vi "ConfigureSsiAbsEncoderSensorType.vi"(4 "error in (no error)":errorcluster, 5 "SSI sensor type":u16(ring)=4 items=["SSI encoder binary coded"=4, "SSI encoder grey coded"=5], 6 "SSI encoder configuration":T1, 7 "axis in":cluster{"keyHandle":u32, "nodeId":u16}={"keyHandle"=0, "nodeId"=1}) -> (0 "error out":errorcluster, 3 "axis out":cluster{"keyHandle":u32, "nodeId":u16}={"keyHandle"=0, "nodeId"=1})   [LabVIEW 2018]
doc: "<B>ConfigureSsiAbsEncoderSensorType</B> writes the value for sensor type 'SSI encoder binary coded' to the device. Parameters from the sensor type can be set."
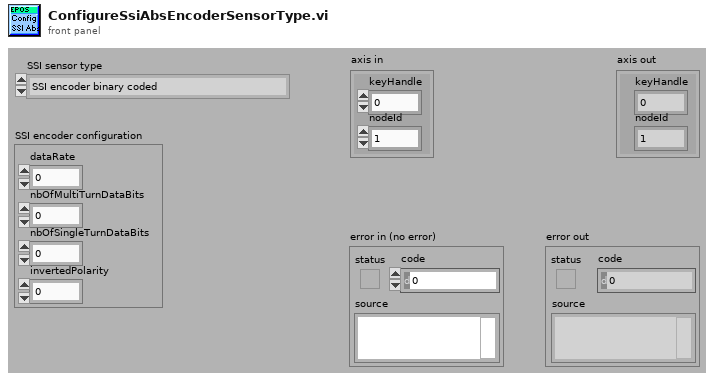
[diagram p1: front panel]
types:
  T1 = cluster{"dataRate":u16, "nbOfMultiTurnDataBits":u16, "nbOfSingleTurnDataBits":u16, "invertedPolarity":i32}
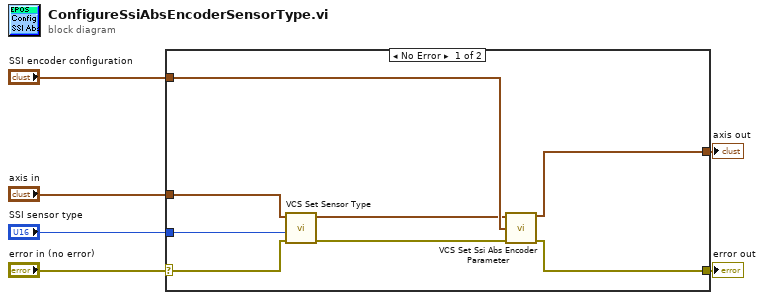
[diagram p0: block diagram]
diagram:
  n1 = case shown="No Error" "error in (no error)" {
    selector: "error in (no error)" -> [w13 w16]
    tunnel: [w11 w16] -> w5
    tunnel: [w10 w15] -> w4
    tunnel: "axis in" -> [w14 w15]
    tunnel: "SSI sensor type" -> [w12 _]
    tunnel: "SSI encoder configuration" -> [w9 _]
    frame No Error {
      n2 = call "VCS Set Sensor Type.vi"("error in (no error)"=w13, "SensorType"=w12, "axis in"=w14) -> ("error out"=w7:errorcluster, "axis out"=w8:cluster{"keyHandle":u32, "nodeId":u16})  [unwired: 7 in]
      n3 = call "VCS Set Ssi Abs Encoder Parameter.vi"("axis in"=w8, "SSI encoder"=w9, "error in (no error)"=w7) -> ("axis out"=w10:cluster{"keyHandle":u32, "nodeId":u16}, "error out"=w11:errorcluster)  [unwired: 11 in]
    }
    frame Error {
    }
  }
  "error out" <- w5
  "axis out" <- w4
